vi "Delete Item By Name.vi"(8 "error in (no error)":errorcluster, 10 "Name":string, 11 "Parent Ref in":T1 format="%.0x") -> (0 "error out":errorcluster, 3 "Parent Ref out":T1 format="%.0x")   [LabVIEW 2015, in "Chassis TimeSync System Explorer.lvlib"]
uses:
  Chassis TimeSync System Explorer.lvlib
  <vilib>/NI Veristand/Custom Device API/Custom Device Item Ref.ctl
  <vilib>/NI Veristand/Custom Device Tools/Custom Device Utility Library/Custom Device Utility Library.lvlib
  <vilib>/NI Veristand/Custom Device API/Custom Device API.lvlib
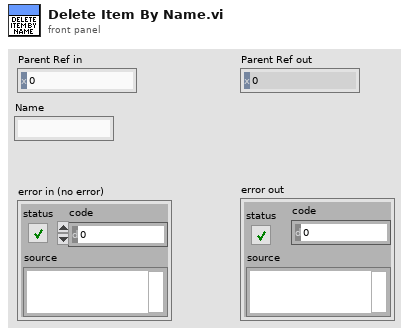
[diagram p1: front panel]
types:
  T1 = typedef "Custom Device API.lvlib/Custom Device Item Ref.ctl" = u64
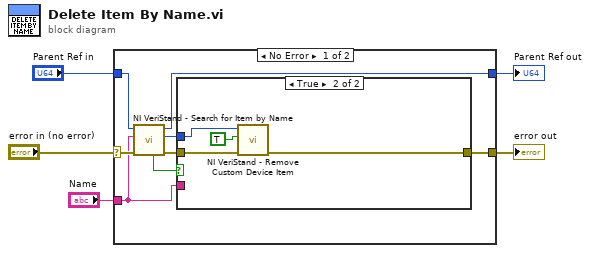
[diagram p0: block diagram]
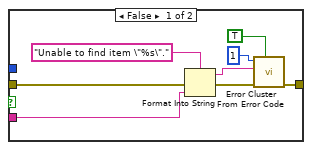
[diagram p2: hidden frame]
diagram:
  n1 = case shown="No Error" "error in (no error)" {
    selector: "error in (no error)" -> [w9 w27]
    tunnel: "Parent Ref in" -> [w11 w26]
    tunnel: [w8 w27] -> w3
    tunnel: [w7 w26] -> w2
    tunnel: "Name" -> [w6 _]
    frame No Error {
      n2 = call <vilib>:"NI VeriStand - Search for Item by Name.vi"("error in"=w9, "Item Name"=w6, "Section Ref in"=w11) -> ("error out"=w10:errorcluster, "Item Ref"=w12:T1, "Section Ref out"=w7:T1, "Found"=w13:bool)  [unwired: 5 in]
      n3 = case shown="True" w13 {
        tunnel: w12 -> [_ w24]
        tunnel: w10 -> [w19 w23]
        tunnel: [w21 w22] -> w8
        tunnel: w6 -> [w16 _]
        frame False {
          n4 = Format Into String(format string="Unable to find item \"%s\"." ("error message (\"\")"), error in=w19, w16) -> (resulting string=w18:string, error out=w17:errorcluster)  [unwired: 1 in]
          n5 = call <vilib>:"Error Cluster From Error Code.vi"("show call chain? (False)"=TRUE, "error in (no error)"=w17, "error message (\"\")"=w18, "error code (0)"=1) -> ("error out"=w21:errorcluster)  [unwired: 5 in]
        }
        frame True {
          n6 = call <vilib>:"NI VeriStand - Remove Custom Device Item.vi"("error in (no error)"=w23, "Force Delete (F)"=TRUE ("Force Rename (F)"), "Item Ref in"=w24) -> ("error out"=w22:errorcluster)  [unwired: 7 in, 1 out]
        }
      }
    }
    frame Error {
    }
  }
  "error out" <- w3
  "Parent Ref out" <- w2
